vi "table_list.vi"(8 "error in (no error)":errorcluster, 11 "toml in":refnum<class "toml.lvclass">) -> (0 "error out":errorcluster, 2 "tables":string[](array[string]), 3 "toml out":refnum<class "toml.lvclass">)   [LabVIEW 2020, in "toml.lvclass"]
doc: "Will create a new table if a table with the same name doesn't already exist"
uses:
  toml.lvclass
  toml.lvclass/toml.ctl
  Doc/Doc.lvclass
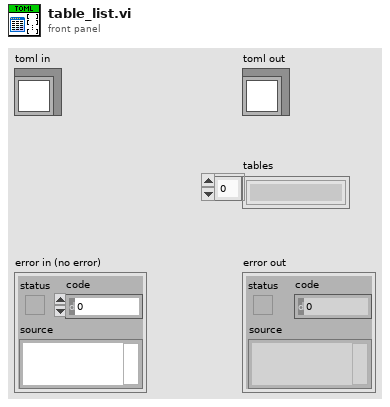
[diagram p1: front panel]
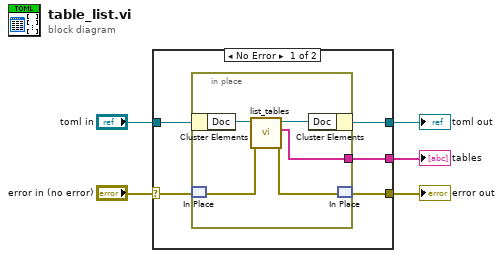
[diagram p0: block diagram]
diagram:
  n1 = case shown="No Error" "error in (no error)" {
    selector: "error in (no error)" -> [w8 w17]
    tunnel: [w7 w17] -> w4
    tunnel: [w9 w16] -> w2
    tunnel: "toml in" -> [w10 w16]
    tunnel: [w6 _] -> w1
    frame No Error {
      n2 = in-place {
        in-place-border: [w11] -> w6
        n3 = in-place-cluster #1(w10) -> ("Doc"=w15:refnum<class "Doc.lvclass">)
        n4 = in-place-match #2(w8) -> (w14:errorcluster)
        n5 = call "list_tables.vi"("error in (no error)"=w14, "Doc in"=w15) -> ("error out"=w12:errorcluster, "table_names"=w11:string[], "Doc out"=w13:refnum<class "Doc.lvclass">)  [unwired: 7 in]
        n6 = in-place-cluster #1("Doc"=w13) -> (w9:refnum<class "toml.lvclass">)
        n7 = in-place-match #2(w12) -> (w7:errorcluster)
      }
    }
    frame Error {
    }
  }
  "error out" <- w4
  "toml out" <- w2
  "tables" <- w1
